vi "MIDI Meta Events scripting.vi"   [LabVIEW 2020]
uses:
  <vilib>/Utility/traverseref.llb/TRef TravTarget.ctl
  midi-file/MIDI Meta Events.ctl
  midi-file/midi-file.lvclass
types:
  T1 = typedef "TRef TravTarget.ctl" = enum16{"FP", "BD", "Other"}
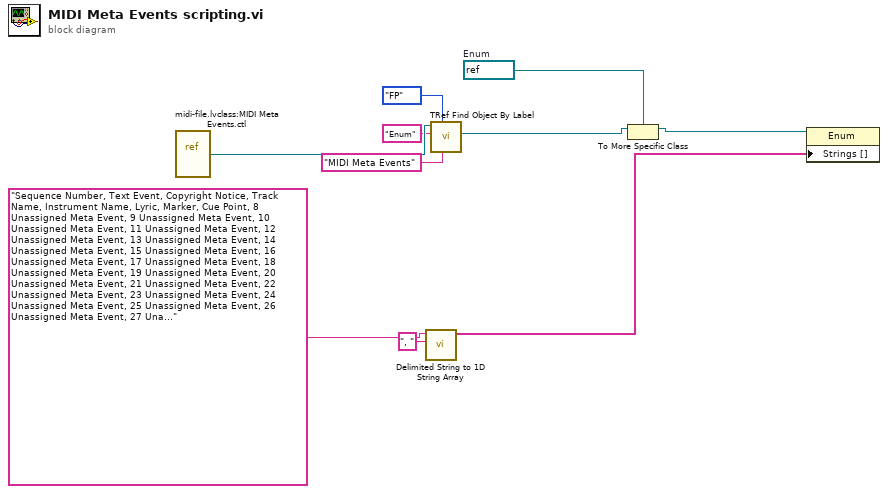
[diagram p0: block diagram]
diagram:
  w5 = refnum<vi> refnum  # Enum
  n1 = vi-ref "midi-file.lvclass:MIDI Meta Events.ctl"() -> (w10:refnum<vi>)
  n2 = call <vilib>:"Delimited String to 1D String Array.vi"("delimiter"=", ", "delimited string"="Sequence Number, Text Event, Copyright Notice, Track Name, Instrument Name, Lyric, Marker, Cue Point, 8 Unassigned Meta Event, 9 Unassigned Meta Event, 10 Unassigned Meta Event, 11 Unassigned Meta Event, 12 Unassigned Meta Event, 13 Unassigned Meta Event, 14 Unassigned Meta Event, 15 Unassigned Meta Event, 16 Unassigned Meta Event, 17 Unassigned Meta Event, 18 Unassigned Meta Event, 19 Unassigned Meta Event, 20 Unassigned Meta Event, 21 Unassigned Meta Event, 22 Unassigned Meta Event, 23 Unassigned Meta Event, 24 Unassigned Meta Event, 25 Unassigned Meta Event, 26 Unassigned Meta Event, 27 Unassigned Meta Event, 28 Unassigned Meta Event, 29 Unassigned Meta Event, 30 Unassigned Meta Event, 31 MIDI Channel Prefix, 32 Unassigned Meta Event, 33 Unassigned Meta Event, 34 Unassigned Meta Event, 35 Unassigned Meta Event, 36 Unassigned Meta Event, 37 Unassigned Meta Event, 38 Unassigned Meta Event, 39 Unassigned Meta Event, 40 Unassigned Meta Event, 41 Unassigned Meta Event, 42 Unassigned Meta Event, 43 Unassigned Meta Event, 44 Unassigned Meta Event, 45 Unassigned Meta Event, 46 Unassigned Meta Event, 47 End of Track, 48 Unassigned Meta Event, 49 Unassigned Meta Event, 50 Unassigned Meta Event, 51 Unassigned Meta Event, 52 Unassigned Meta Event, 53 Unassigned Meta Event, 54 Unassigned Meta Event, 55 Unassigned Meta Event, 56 Unassigned Meta Event, 57 Unassigned Meta Event, 58 Unassigned Meta Event, 59 Unassigned Meta Event, 60 Unassigned Meta Event, 61 Unassigned Meta Event, 62 Unassigned Meta Event, 63 Unassigned Meta Event, 64 Set Tempo, 65 Unassigned Meta Event, 66 Unassigned Meta Event, 67 Unassigned Meta Event, 68 SMPTE Offset, 69 Unassigned Meta Event, 70 Unassigned Meta Event, 71 Unassigned Meta Event, 72 Unassigned Meta Event, 73 Time Signature, 74 Key Signature, 75 Unassigned Meta Event, 76 Unassigned Meta Event, 77 Unassigned Meta Event, 78 Unassigned Meta Event, 79 Unassigned Meta Event, 80 Unassigned Meta Event, 81 Unassigned Meta Event, 82 Unassigned Meta Event, 83 Unassigned Meta Event, 84 Unassigned Meta Event, 85 Unassigned Meta Event, 86 Unassigned Meta Event, 87 Unassigned Meta Event, 88 Unassigned Meta Event, 89 Unassigned Meta Event, 90 Unassigned Meta Event, 91 Unassigned Meta Event, 92 Unassigned Meta Event, 93 Unassigned Meta Event, 94 Unassigned Meta Event, 95 Unassigned Meta Event, 96 Unassigned Meta Event, 97 Unassigned Meta Event, 98 Unassigned Meta Event, 99 Unassigned Meta Event, 100 Unassigned Meta Event, 101 Unassigned Meta Event, 102 Unassigned Meta Event, 103 Unassigned Meta Event, 104 Unassigned Meta Event, 105 Unassigned Meta Event, 106 Unassigned Meta Event, 107 Unassigned Meta Event, 108 Unassigned Meta Event, 109 Unassigned Meta Event, 110 Unassigned Meta Event, 111 Unassigned Meta Event, 112 Unassigned Meta Event, 113 Unassigned Meta Event, 114 Unassigned Meta Event, 115 Unassigned Meta Event, 116 Unassigned Meta Event, 117 Unassigned Meta Event, 118 Unassigned Meta Event, 119 Unassigned Meta Event, 120 Unassigned Meta Event, 121 Unassigned Meta Event, 122 Unassigned Meta Event, 123 Unassigned Meta Event, 124 Unassigned Meta Event, 125 Unassigned Meta Event, 126 Unassigned Meta Event, 127 Sequencer-Specific Meta Event" ("Label")) -> ("string array"=w1:string[])  [unwired: 9 in]
  n3 = call <vilib>:"TRef Find Object By Label.vi"("Label"="MIDI Meta Events", "Traverse Target"=TRef_TravTarget."FP", "Class Name"="Enum", "VI Ref"=w10) -> ("Found Obj Ref"=w6:refnum<vi>)  [unwired: 4 in, 3 out]
  n4 = To More Specific Class(target class=w5, reference=w6) -> (specific class reference=w4:refnum<vi>)  [unwired: 1 in, 1 out]
  n5 = property class="Enum"(reference=w4, "Strings []"=w1) -> ()  [unwired: 1 in, 2 out]
